vi "Set Controller Configuration.vi"(8 "error in (no error)":errorcluster, 11 "Controller in":refnum<class "Controller.lvclass">) -> (0 "error out":errorcluster, 3 "Controller out":refnum<class "Controller.lvclass">)   [LabVIEW 2016, in "Controller Actor.lvlib" / "Controller.lvclass"]
uses:
  <userlib>/Common Components/Controller/Controller.lvclass
  <userlib>/Common Components/FCN Configuration/Controller Configuration.lvclass
  <vilib>/Utility/sysdir.llb/System Directory Type.ctl
  <userlib>/Common Components/Controller/Controller.lvclass/Controller.ctl
  <userlib>/Common Components/FCN Configuration/Controller Configuration.lvclass/Controller Configuration.ctl
  <userlib>/Common Components/FCN Configuration/Read HW Paths.vi
  <userlib>/Common Components/FCN Configuration/Read FindHardwareInAppData.vi
  <userlib>/Common Components/FCN Configuration/Read Fcn Paths.vi
  <userlib>/Common Components/FCN Configuration/Read FindFunctionsInAppData.vi
  <userlib>/Configuration Dialog Actor/Configuration.lvclass
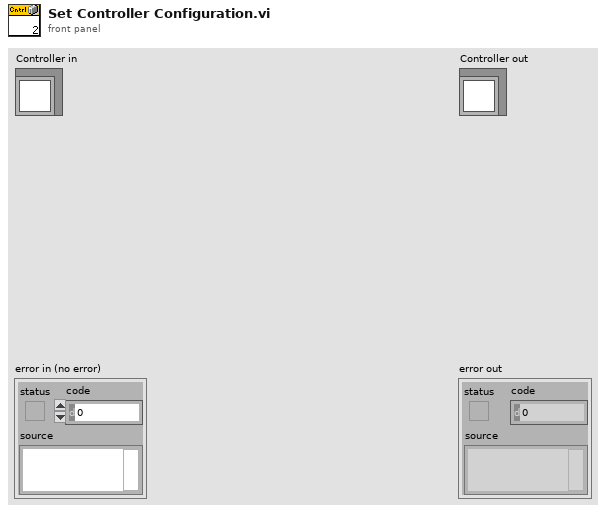
[diagram p1: front panel]
types:
  T1 = typedef "System Directory Type.ctl" = i32
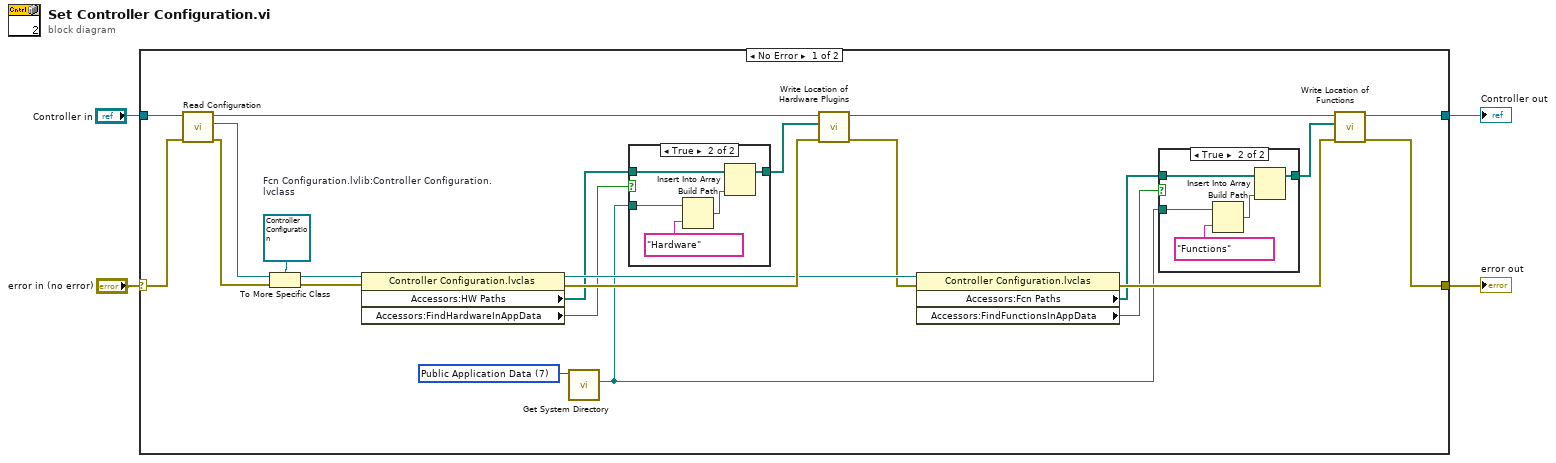
[diagram p0: block diagram]
diagram:
  n1 = case shown="No Error" "error in (no error)" {
    selector: "error in (no error)" -> [w25 w41]
    tunnel: [w5 w41] -> w3
    tunnel: [w6 w40] -> w1
    tunnel: "Controller in" -> [w27 w40]
    frame No Error {
      w18 = T1 7 items=["User Home"=0, "User Desktop"=1, "User Documents"=2, "User Application Data"=3, "User Preferences"=4, "User Temporary"=5, "Public Documents"=6, "Public Application Data"=7, "Public Preferences"=8, "Public Cache"=13, "System Core Libraries"=9, "System Installed Libraries"=10, "Application Files"=11, "Boot Volume Root"=12] ("system directory type")
      w23 = refnum<class "Controller Configuration.lvclass"> refnum  # Fcn Configuration.lvlib:Controller Configuration.lvclass
      n2 = call <userlib>:"Read Configuration.vi"("error in (no error)"=w25, "Controller in"=w27) -> ("error out"=w22:errorcluster, "Configuration.lvlib:Configuration.lvclass"=w21:refnum<class "Configuration.lvclass">, "Controller out"=w26:refnum<class "Controller.lvclass">)  [unwired: 7 in]
      n3 = To More Specific Class(target class=w23, reference=w21, error in=w22) -> (specific class reference=w8:refnum<class "Controller Configuration.lvclass">, error out=w7:errorcluster)
      n4 = property class="Controller Configuration.lvclas"(reference=w8, error in=w7) -> (reference out=w20:refnum<class "Controller Configuration.lvclass">, error out=w24:errorcluster, "Accessors:HW Paths"=w17:path[], "Accessors:FindHardwareInAppData"=w15:bool)
      n5 = call <vilib>:"Get System Directory.vi"("system directory type"=w18) -> ("system directory"=w12:path)  [unwired: 10 in]
      n6 = case shown="True" w15 {
        tunnel: w17 -> [w34 w39]
        tunnel: [w34 w38] -> w16
        tunnel: w12 -> [_ w36]
        frame False {
        }
        frame True {
          n7 = Build Path(base path=w36, name or relative path="Hardware") -> (appended path=w37:path)
          n8 = Insert Into Array(array=w39, new element=w37) -> (w38:path[])  [unwired: 1 in]
        }
      }
      n9 = call <userlib>:"Write Location of Hardware Plugins.vi"("error in (no error)"=w24, "Array of Hardware Paths"=w16, "Controller in"=w26) -> ("error out"=w9:errorcluster, "Controller out"=w10:refnum<class "Controller.lvclass">)  [unwired: 7 in]
      n10 = property class="Controller Configuration.lvclas"(reference=w20, error in=w9) -> (error out=w19:errorcluster, "Accessors:Fcn Paths"=w14:path[], "Accessors:FindFunctionsInAppData"=w13:bool)  [unwired: 1 out]
      n11 = case shown="True" w13 {
        tunnel: w14 -> [w28 w33]
        tunnel: [w28 w32] -> w11
        tunnel: w12 -> [_ w30]
        frame False {
        }
        frame True {
          n12 = Build Path(base path=w30, name or relative path="Functions") -> (appended path=w31:path)
          n13 = Insert Into Array(array=w33, new element=w31) -> (w32:path[])  [unwired: 1 in]
        }
      }
      n14 = call <userlib>:"Write Location of Functions.vi"("error in (no error)"=w19, "Array of Functions"=w11, "UI Controller in"=w10) -> ("error out"=w5:errorcluster, "UI Controller out"=w6:refnum<class "Controller.lvclass">)  [unwired: 7 in]
    }
    frame Error {
    }
  }
  "error out" <- w3
  "Controller out" <- w1
